vi "Min Read Single.vi"(8 "error in":errorcluster, 9 "Channel Index":i32=1, 11 "Min Power Limit in":refnum<class "Power Limit.lvclass">) -> (0 "error out":errorcluster, 1 "Changed or First Call?":bool, 2 "Power Min SP":dbl, 3 "Min Power Limit out":refnum<class "Power Limit.lvclass">)   [LabVIEW 2023, in "Power Limit.lvclass"]
uses:
  Power Limit.lvclass
  Power Limit.lvclass/Power Limit.ctl
  Parents/Limit/Limit.lvclass
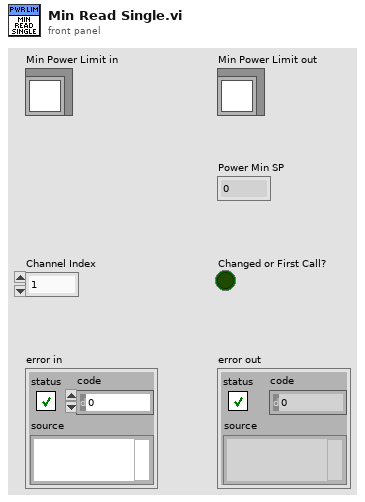
[diagram p1: front panel]
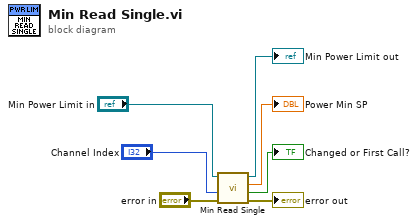
[diagram p0: block diagram]
diagram:
  n1 = call-parent "Min Read Single.vi"("error in"="error in", "Channel Index"="Channel Index", "Min Limit in"="Min Power Limit in") -> ("error out"=→"error out":errorcluster, "Changed or First Call?"=→"Changed or First Call?":bool, "Current Min SP"=→"Power Min SP":dbl, "Min Limit out"=→"Min Power Limit out":refnum<class "Power Limit.lvclass">)  [unwired: 5 in]
